vi "SVT Shock Response Spectrum (1 Ch - 1 Max Type).vi"(0 "scaled signal [EU]":waveform(dbl), 1 "maximum value type":i32(ring) items=["Maximax", "Initial positive", "Initial negative", "Initial absolute", "Residual positive", "Residual negative", "Residual absolute"], 2 "pulse duration [ms]":dbl=-1.0 format="%.2f", 5 "frequency range":T2={"low frequency [Hz]"=10.0, "high frequency [Hz]"=100.0, "frequencies / octave"=6} {"high frequency [Hz]" format="%.2f"; "low frequency [Hz]" format="%.2f"}, 7 "model":i32(ring) items=["Absolute acceleration", "Relative displacement"], 9 "critical damping factor":dbl=0.05 format="%.2f", 11 "error in (no error)":errorcluster, 12 "preprocessing settings":T3 {"lowpass cutoff frequency [Hz]" format="%.2f"}, 13 "desired units":i32(ring)=-1 items=["no change"=-1, "m/s^2"=0, "mm/s^2"=2, "micron/s^2"=3, "in/s^2"=1, "mil/s^2"=5]) -> (4 "shock spectrum":T1 {"maximum values" format="%.2f"; "natural frequencies [Hz]" format="%.2f"}, 6 "unit label":string, 15 "error out":errorcluster)   [LabVIEW 2017, in "SoundVib_Transient.lvlib"]
doc: "Computes the peak levels for each single-degree-of-freedom (SDOF) component to form the shock response spectrum (SRS) across the <B>frequency range</B> of interest. Wire data to the <B>scaled signal [EU]</B> input to determine the polymorphic instance to use or manually select the instance."
uses:
  <vilib>/addons/Sound and Vibration/svt_Transients/SoundVib_Transient.lvlib
  <vilib>/addons/_NISVFA/_Shared subVIs/Common/svc_Engineering Units to Unit Label.vi
  <vilib>/addons/_NISVFA/_Shared subVIs/Common/svc_Unit Label to Engineering Units.vi
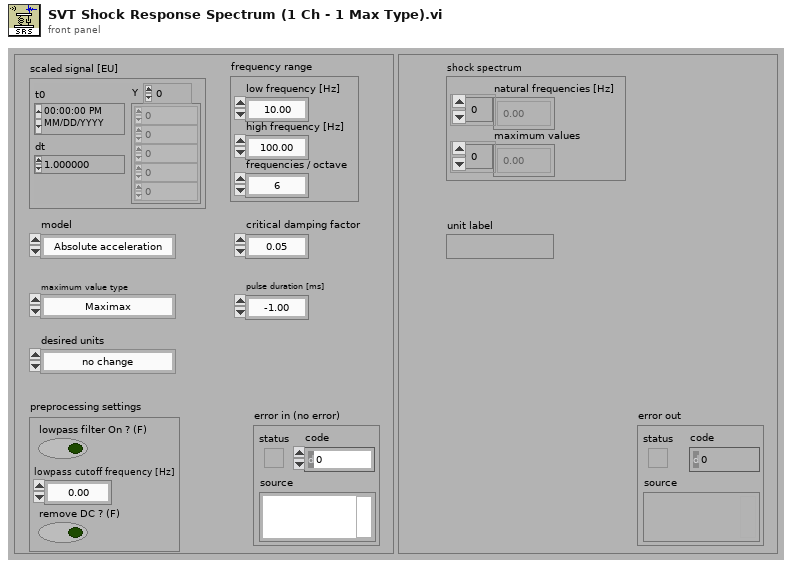
[diagram p1: front panel]
types:
  T1 = cluster{"natural frequencies [Hz]":dbl[], "maximum values":dbl[]}
  T2 = cluster{"low frequency [Hz]":dbl, "high frequency [Hz]":dbl, "frequencies / octave":i32}
  T3 = cluster{"lowpass filter On ? (F)":bool, "lowpass cutoff frequency [Hz]":dbl, "remove DC ? (F)":bool}
  T4 = cluster{"natural frequencies [Hz]":dbl[], "scaled array":dbl[]}
  T5 = typedef "svc_Channel Info.ctl" = cluster{"sensor sensitivity":dbl, "engineering units":T6, "dB reference":dbl, "custom label":string, "weighting filter":T7, "pregain":dbl}
  T6 = typedef "svc_Engineering Units Text Ring.ctl" = u16
  T7 = typedef "svc_Weighting Filter Text Ring.ctl" = u16
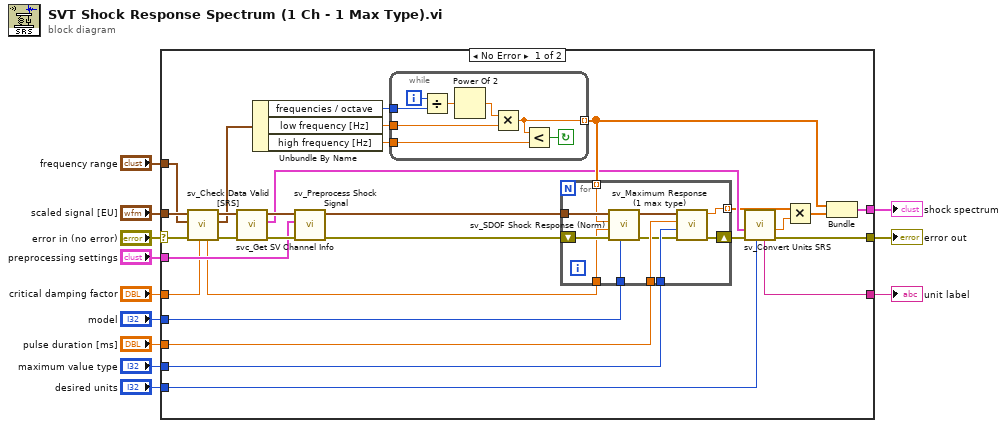
[diagram p0: block diagram]
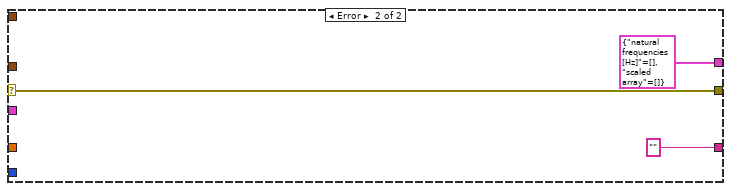
[diagram p2: hidden frame]
diagram:
  n1 = case shown="No Error" "error in (no error)" {
    selector: "error in (no error)" -> [w28 w63]
    tunnel: [w20 w63] -> w11
    tunnel: "scaled signal [EU]" -> [w32 _]
    tunnel: "preprocessing settings" -> [w34 _]
    tunnel: "frequency range" -> [w29 _]
    tunnel: "pulse duration [ms]" -> [w39 _]
    tunnel: [w38 T4 {"natural frequencies [Hz]"=[], "scaled array"=[]}] -> w2
    tunnel: "critical damping factor" -> [w26 _]
    tunnel: "model" -> [w37 _]
    tunnel: "maximum value type" -> [w33 _]
    tunnel: [w15 "" ("unit label")] -> w4
    tunnel: "desired units" -> [w19 _]
    frame No Error {
      n2 = call <vilib>:"sv_Check Data Valid [SRS].vi"("critical damping factor"=w26, "error in (no error)"=w28, "frequency range"=w29, "scaled signal [EU]"=w32) -> ("error out"=w30:errorcluster, "dup frequency range"=w13:T2, "dup scaled signal [EU]"=w31:waveform(dbl), "dup critical damping"=w27:dbl)  [unwired: 4 in]
      n3 = call <vilib>:"svc_Get SV Channel Info.vi"("error in (no error)"=w30, "scaled signal [EU]"=w31) -> ("error out"=w35:errorcluster, "channel info"=w18:T5, "dup scaled signal [EU]"=w36:waveform(dbl))  [unwired: 4 in, 3 out]
      n4 = Unbundle By Name(w13) -> ("frequencies / octave"=w23:i32, "low frequency [Hz]"=w24:dbl, "high frequency [Hz]"=w25:dbl)
      n5 = call <vilib>:"sv_Preprocess Shock Signal.vi"("error in (no error)"=w35, "preprocessing settings"=w34, "scaled signal [EU]"=w36) -> ("error out"=w40:errorcluster, "filtered scaled signal [EU]"=w41:waveform(dbl))  [unwired: 7 in]
      n6 = while {
        tunnel: [w42] -> w22 mode=indexing
        tunnel: w25 -> [w44]
        tunnel: w24 -> [w45]
        tunnel: w23 -> [w48]
        i -> [w49]
        stop <- w43 continue-if-true
        n7 = Divide(x=w49, y=w48) -> (x/y=w47:dbl)
        n8 = Power Of 2(x=w47) -> (2^x=w46:dbl)
        n9 = Multiply(x=w46, y=w45) -> (x*y=w42:dbl)
        n10 = Less?(x=w42, y=w44) -> (x < y?=w43:bool)
      }
      n11 = for {
        tunnel: w41 -> [w56]
        tunnel: w27 -> [w54]
        tunnel: w33 -> [w60]
        tunnel: [w58] -> w17 mode=indexing
        tunnel: w37 -> [w53]
        shift-right: [w59] -> w21
        shift-left: w40 -> [w55]
        tunnel: w39 -> [w57]
        tunnel: w22 -> [w50] mode=indexing
        n12 = call <vilib>:"sv_SDOF Shock Response (Norm).vi"("model"=w53, "error in (no error)"=w55, "critical damping factor"=w54, "fn [Hz]"=w50, "scaled signal [EU]"=w56) -> ("error out"=w51:errorcluster, "SDOF shock response"=w52:waveform(dbl))  [unwired: 5 in]
        n13 = call <vilib>:"sv_Maximum Response (1 max type).vi"("error in (no error)"=w51, "maximum value type"=w60, "pulse duration [ms]"=w57, "SDOF shock response"=w52) -> ("error out"=w59:errorcluster, "maximum value"=w58:dbl)  [unwired: 4 in, 2 out]
      }
      n14 = call <vilib>:"sv_Convert Units SRS.vi"("desired units"=w19, "error in (no error)"=w21, "channel info"=w18) -> ("error out"=w20:errorcluster, "scale factor"=w14:dbl, "unit label"=w15:string)  [unwired: 4 in]
      n15 = Multiply(x=w17, y=w14) -> (x*y=w16:dbl[])
      n16 = Bundle(w22, w16) -> (w38:cluster{dbl[], dbl[]})  [unwired: 1 in]
    }
    frame Error {
    }
  }
  "error out" <- w11
  "unit label" <- w4
  "shock spectrum" <- w2
